vi "RT Watchdog.vi"(8 "error in (no error)":errorcluster, 10 "info":cluster{"File path":T1, "Cfg ":T2} {"Cfg"."Offset_rueda WS 2" format="%.27g"; "Cfg"."Offset_rueda WS 1" format="%.27g"; "Cfg"."Frecuencia de muestreo y módulo CRIO" items=["51.200 kS/s (NI 9234)"=1, "25.600 kS/s (NI 9234)"=2, "17.067 kS/s (NI 9234)"=3, "12.800 kS/s (NI 9234)"=4, "10.240 kS/s (NI 9234)"=5, "8.533 kS/s (NI 9234)"=6, "7.314 kS/s (NI 9234)"=7, "6.400 kS/s (NI 9234)"=8, "5.689 kS/s (NI 9234)"=9, "5.120 kS/s (NI 9234)"=10, "4.654 kS/s (NI 9234)"=11, "4.267 kS/s (NI 9234)"=12, "3.938 kS/s (NI 9234)"=13, "3.657 kS/s (NI 9234)"=14, "3.413 kS/s (NI 9234)"=15, "3.200 kS/s (NI 9234)"=16, "3.012 kS/s (NI 9234)"=17, "2.845 kS/s (NI 9234)"=18, "2.695 kS/s (NI 9234)"=19, "2.560 kS/s (NI 9234)"=20, "2.438 kS/s (NI 9234)"=21, "2.328 kS/s (NI 9234)"=22, "2.226 kS/s (NI 9234)"=23, "2.133 kS/s (NI 9234)"=24, "2.048 kS/s (NI 9234)"=25, "1.969 kS/s (NI 9234)"=26, "1.896 kS/s (NI 9234)"=27, "1.829 kS/s (NI 9234)"=28, "1.765 kS/s (NI 9234)"=29, "1.707 kS/s (NI 9234)"=30, "1.652 kS/s (NI 9234)"=31]}, 11 "Message Queues in":T4) -> (0 "error out":errorcluster)   [LabVIEW 2015]
uses:
  support/Message Queue/All Message Queues.ctl
  support/Message Queue/Message Cluster.ctl
  controls/File paths.ctl
  controls/Cfg_parameters.ctl
  <vilib>/LabVIEW Targets/FPGA/cRIO/shared/nicrio_ModuleControls/nicrio_cRIO-9234_DataRatesRing2.ctl
  <vilib>/RTwatchdog.llb/Watchdog expiration actions.ctl
  support/Message Queue/Enqueue Message (Single).vi
  <vilib>/Utility/error.llb/Error Cluster From Error Code.vi
  <vilib>/ErrorRing/Error Ring.xnode
  support/Message Queue/Message Queue.lvlib
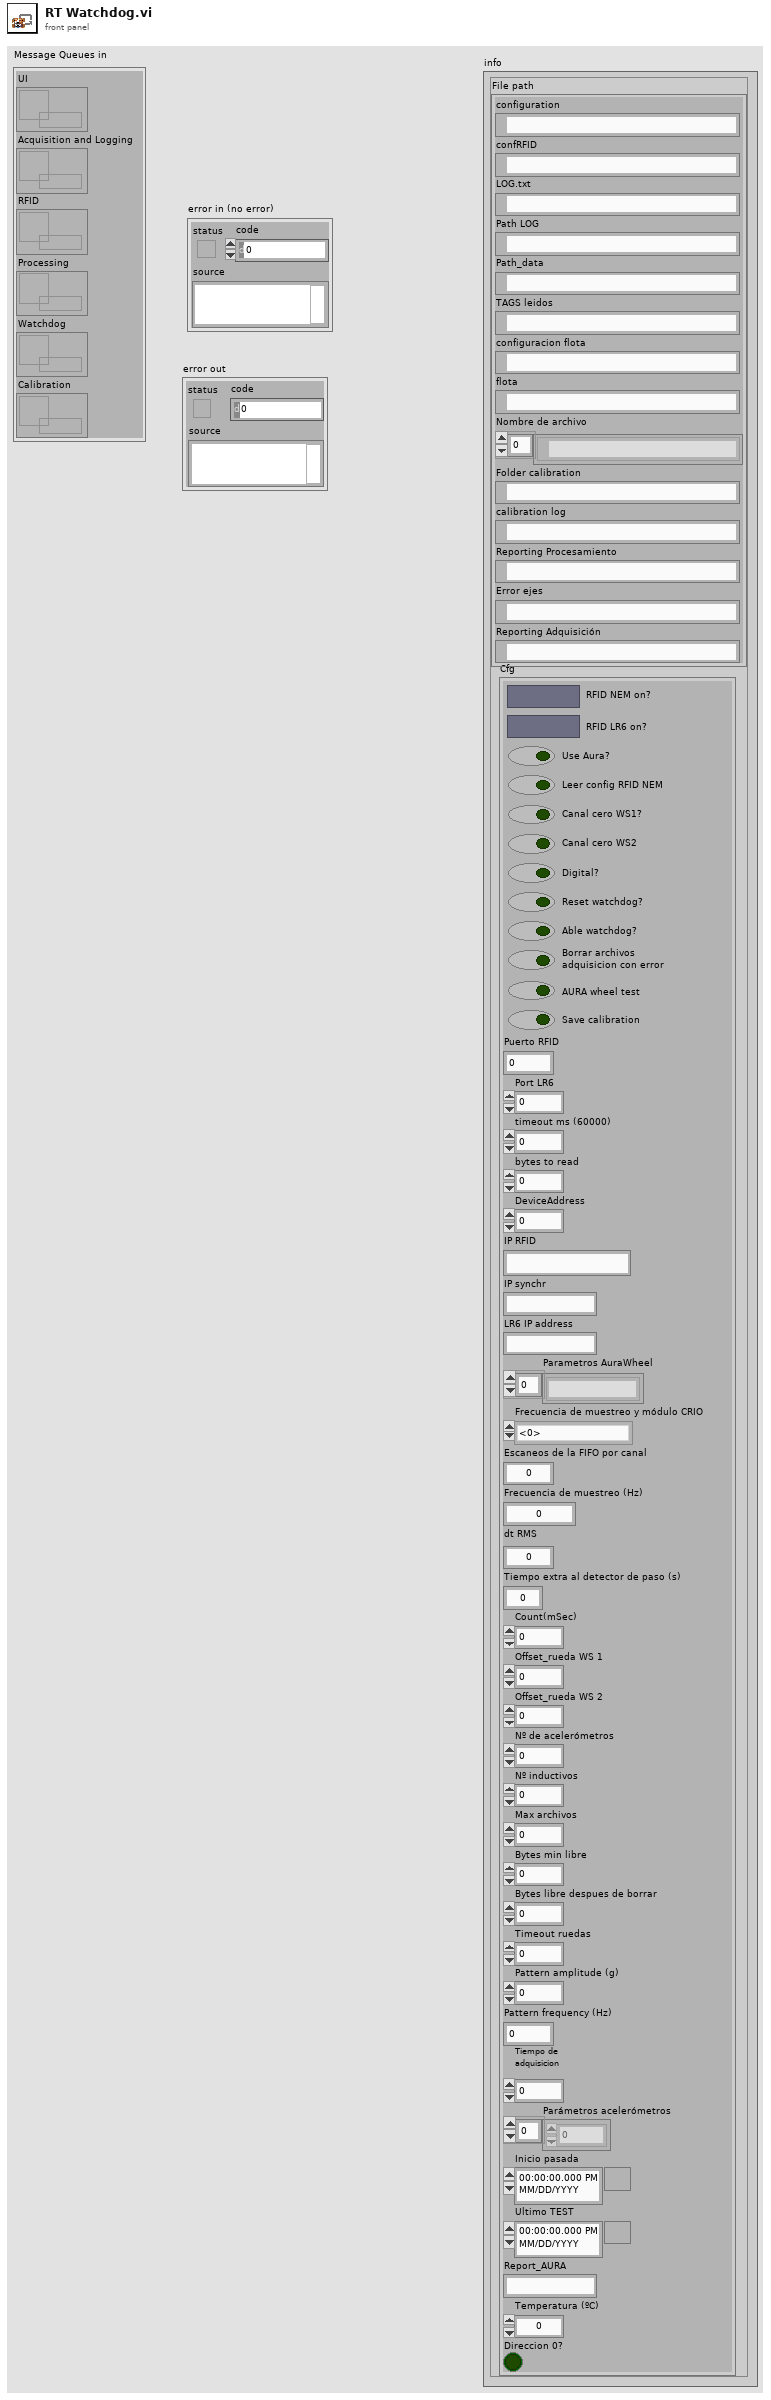
[diagram p1: front panel]
types:
  T1 = typedef "File paths.ctl" = cluster{"configuration":path, "confRFID":path, "LOG.txt":path, "Path LOG":path, "Path_data":path, "TAGS leidos":path, "configuracion flota":path, "flota":path, "Nombre de archivo":path[], "Folder calibration":path, "calibration log":path, "Reporting Procesamiento":path, "Error ejes":path, "Reporting Adquisición":path}
  T2 = typedef "Cfg_parameters.ctl" = cluster{"RFID NEM on?":bool, "RFID LR6 on?":bool, "Use Aura?":bool, "Leer config RFID NEM":bool, "Canal cero WS1?":bool, "Canal cero WS2 ":bool, "Digital?":bool, "Reset watchdog?":bool, "Able watchdog?":bool, "Borrar archivos\nadquisicion con error":bool, "AURA wheel test":bool, "Save calibration":bool, "Puerto RFID":u16, "Port LR6":u16, "timeout ms (60000)":i32, "bytes to read":i32, "DeviceAddress":u8, "IP RFID":string, "IP synchr":string, "LR6 IP address":string, "Parametros AuraWheel":string[], "Frecuencia de muestreo y módulo CRIO":T3, "Escaneos de la FIFO por canal":u32, "Frecuencia de muestreo (Hz)":dbl, "dt RMS":dbl, "Tiempo extra al detector de paso (s)":dbl, "Count(mSec)":u32, "Offset_rueda WS 1":fxp<+/-,24,-4>, "Offset_rueda WS 2":fxp<+/-,24,-4>, "Nº de acelerómetros":i32, "Nº inductivos":i32, "Max archivos":u32, "Bytes min libre":u32, "Bytes libre despues de borrar":u32, "Timeout ruedas":dbl, "Pattern amplitude (g)":dbl, "Pattern frequency (Hz)":dbl, "Tiempo de adquisicion\n":dbl, "Parámetros acelerómetros":dbl[], "Inicio pasada":timestamp, "Ultimo TEST":timestamp, "Report_AURA":string, "Temperatura (ºC)":dbl, "Direccion 0?":bool}
  T3 = typedef "nicrio_cRIO-9234_DataRatesRing2.ctl" = u8
  T4 = typedef "Message Queue.lvlib/All Message Queues.ctl" = cluster{"UI":refnum<queue>, "Acquisition and Logging":refnum<queue>, "RFID":refnum<queue>, "Processing":refnum<queue>, "Watchdog":refnum<queue>, "Calibration":refnum<queue>}
  T5 = typedef "Watchdog expiration actions.ctl" = cluster{"reset":bool, "occurrence":bool, "trigger protocol":enum16{"active high", "active low", "open collector"}, "trigger line":enum16{"none", "line 0", "line 1", "line 2", "line 3", "line 4", "line 5", "line 6", "line 7", "SMB line 0"}, "disable watchdog on VI exit":bool}
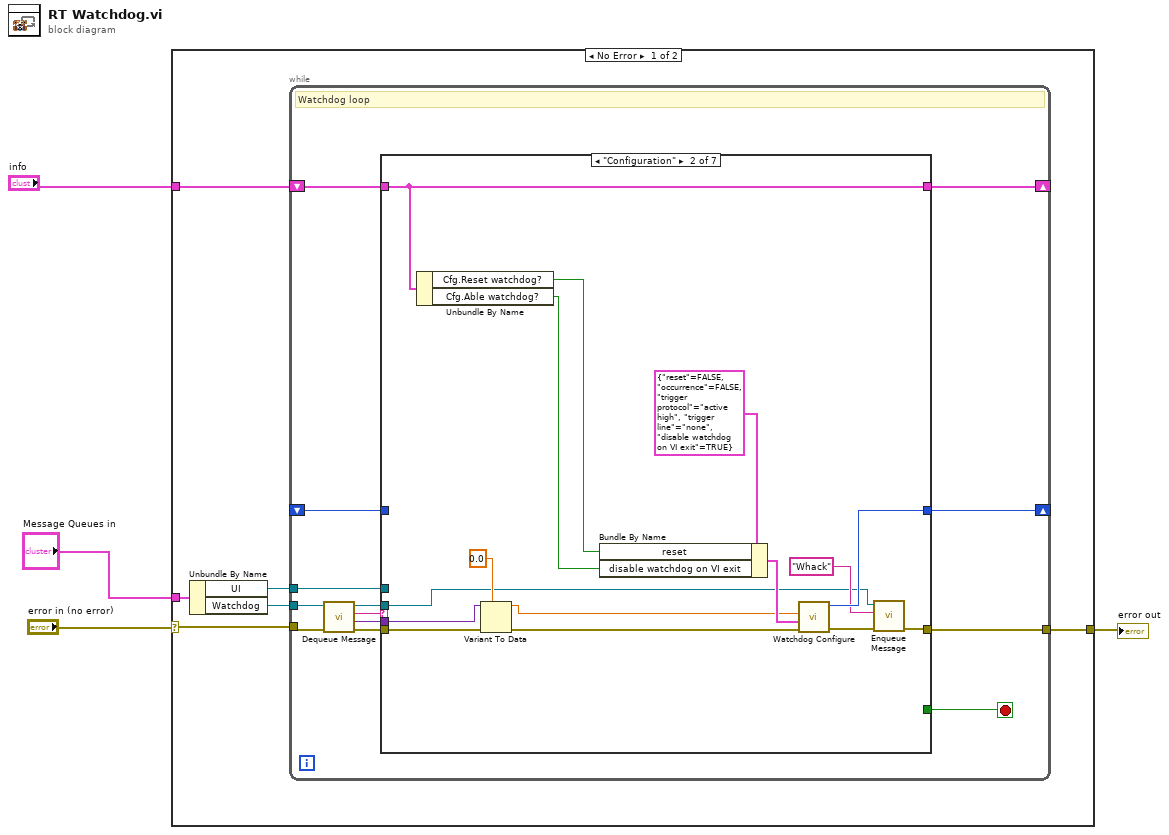
[diagram p0: block diagram]
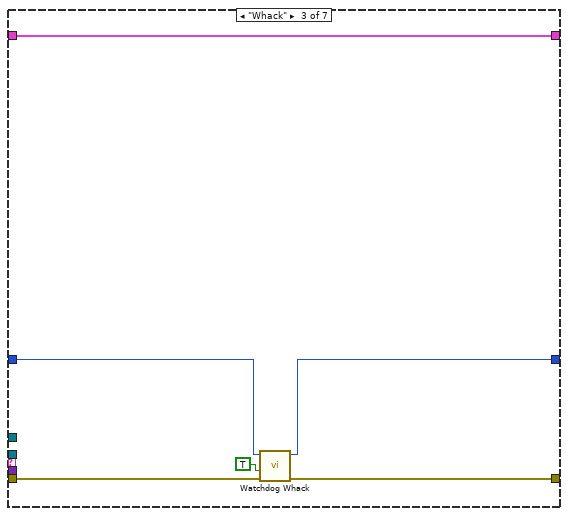
[diagram p3: hidden frame]
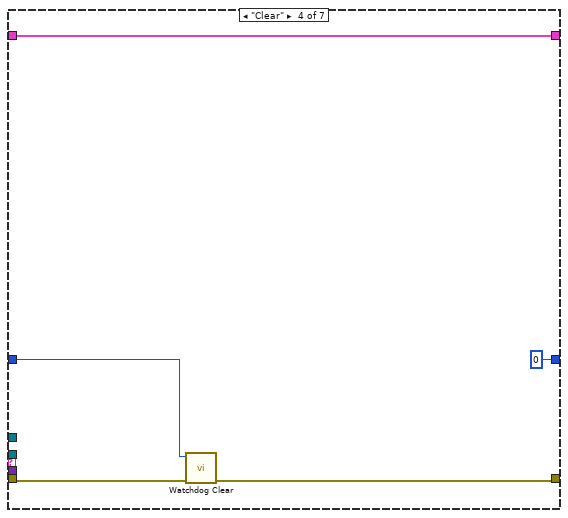
[diagram p4: hidden frame]
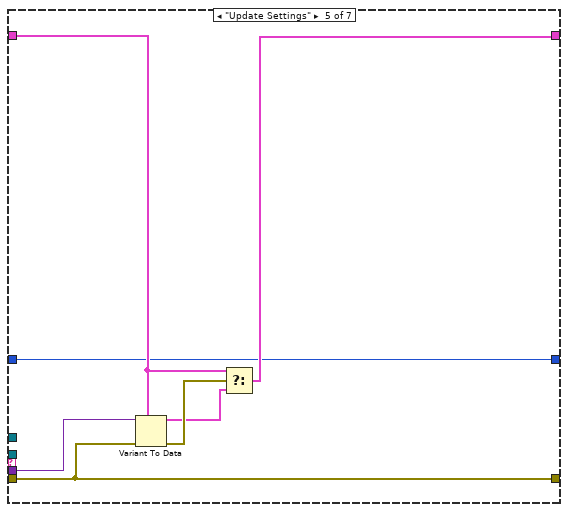
[diagram p5: hidden frame]
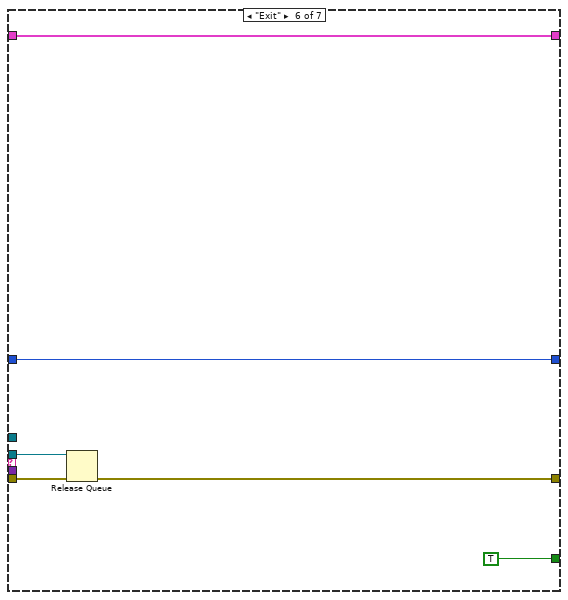
[diagram p6: hidden frame]
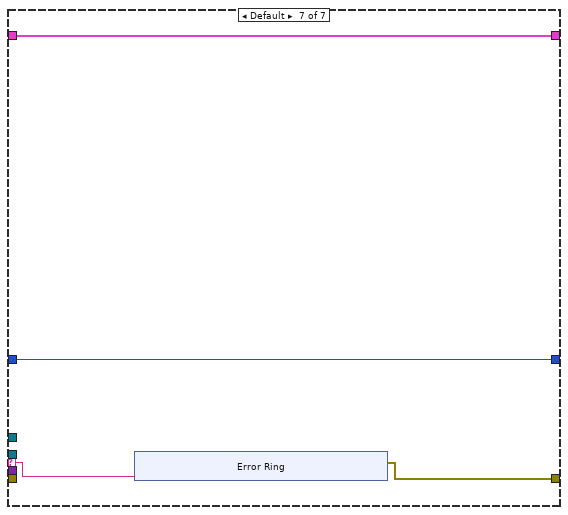
[diagram p7: hidden frame]
diagram:
  n1 = case shown="No Error" "error in (no error)" {
    selector: "error in (no error)" -> [w9 w77]
    tunnel: "Message Queues in" -> [w10 _]
    tunnel: "info" -> [w6 _]
    tunnel: [w5 w77] -> w1
    frame No Error {
      n2 = Unbundle By Name(w10) -> ("UI"=w7:refnum<queue>, "Watchdog"=w8:refnum<queue>)
      n3 = while {
        tunnel: w9 -> [w23]
        tunnel: w8 -> [w22]
        tunnel: w7 -> [w20]
        shift-right: [w16] -> _
        shift-left: w6 -> [w17]
        tunnel: [w14] -> w5
        shift-right: [w12] -> _
        shift-left: _ -> [w11]
        stop <- w15 stop-if-true
        # "Watchdog loop"
        n4 = call "Dequeue Message.vi"("error in (no error)"=w23, "Message Queue"=w22) -> ("error out"=w19:errorcluster, "Message Data"=w13:variant, "Message"=w18:string, "dup Message Queue"=w21:refnum<queue>)  [unwired: 6 in]
        n5 = case shown="\"Configuration\"" w18 {
          selector: w18 -> [_ _ _ _ _ _ w67]
          tunnel: w21 -> [_ w27 _ _ _ w63 _]
          tunnel: w20 -> [_ _ _ _ _ _ _]
          tunnel: w19 -> [w26 w36 w46 w51 w56 w64 _]
          tunnel: [w26 w30 w45 w50 w56 w62 w68] -> w14
          tunnel: w17 -> [w25 w39 w42 w52 w55 w65 w69]
          tunnel: [w25 w39 w42 w52 w54 w65 w69] -> w16
          tunnel: [_ _ _ _ _ TRUE _] -> w15
          tunnel: w13 -> [_ w33 _ _ w59 _ _]
          tunnel: [w24 w32 w43 u64 0 ("watchdogID out") w53 w60 w66] -> w12
          tunnel: w11 -> [w24 _ w44 w49 w53 w60 w66]
          frame "Initialize" {
          }
          frame "Configuration" {
            n6 = Unbundle By Name(w39) -> ("Cfg.Reset watchdog?"=w38:bool, "Cfg.Able watchdog?"=w37:bool)
            n7 = Variant To Data(error in=w36, type=0.0, Variant=w33) -> (data=w29:dbl, error out=w35:errorcluster)
            n8 = Bundle By Name(cluster=T5 {"reset"=FALSE, "occurrence"=FALSE, "trigger protocol"=enum."active high", "trigger line"=enum."none", "disable watchdog on VI exit"=TRUE} ("expiration actions"), "reset"=w38, "disable watchdog on VI exit"=w37) -> (w41:T5)
            n9 = call <vilib>:"Watchdog Configure.vi"("error in (no error)"=w35, "expiration actions"=w41, "timeout (1 sec)"=w29) -> ("error out"=w31:errorcluster, "watchdogID"=w32:u64)  [unwired: 1 in, 2 out]
            n10 = call-poly "Enqueue Message.vi"("error in (no error)"=w31, "Message"="Whack", "Message Queue"=w27) -> ("error out"=w30:errorcluster)  [unwired: 7 in, 1 out]
          }
          frame "Whack" {
            n11 = call <vilib>:"Watchdog Whack.vi"("error in (no error)"=w46, "reset watchdog after expire? (F)"=TRUE, "watchdogID in"=w44) -> ("error out"=w45:errorcluster, "watchdogID out"=w43:u64)  [unwired: 2 in, 1 out]
          }
          frame "Clear" {
            n12 = call <vilib>:"Watchdog Clear.vi"("error in (no error)"=w51, "watchdogID in"=w49) -> ("error out"=w50:errorcluster)  [unwired: 5 in]
          }
          frame "Update Settings" {
            n13 = Variant To Data(error in=w56, type=w55, Variant=w59) -> (data=w57:cluster{"File path":T1, "Cfg ":T2}, error out=w58:errorcluster)
            n14 = Select(t=w55, s=w58, f=w57) -> (s? t:f=w54:cluster{"File path":T1, "Cfg ":T2})
          }
          frame "Exit" {
            n15 = Release Queue(queue=w63, error in (no error)=w64) -> (error out=w62:errorcluster)  [unwired: 1 in, 2 out]
          }
          frame Default {
            n16 = xnode "Error Ring"("parameter 0"=w67) -> ("error out"=w68:errorcluster)
          }
        }
      }
    }
    frame Error {
    }
  }
  "error out" <- w1
